vi "Tipo Señal.vi"(8 "error in (no error)":errorcluster, 10 "Tipo Señal":u16, 11 "F Generator in":refnum<class "F Generator.lvclass">) -> (0 "error out":errorcluster, 3 "F Generator out":refnum<class "F Generator.lvclass">)   [LabVIEW 2020, in "F Generator.lvlib" / "F Generator.lvclass"]
uses:
  F Generator.lvclass
  F Generator.lvclass/F Generator.ctl
  <vilib>/ActorFramework/Message Enqueuer/Message Enqueuer.lvclass/Message Enqueuer.ctl
  <vilib>/ActorFramework/Message Enqueuer/Enqueue.vi
  C:/Program Files/National Instruments/LabVIEW 2020/vi.lib/ActorFramework/Message/Message.lvclass
  <vilib>/ActorFramework/Message Priority Queue/Priority Enqueue.vi
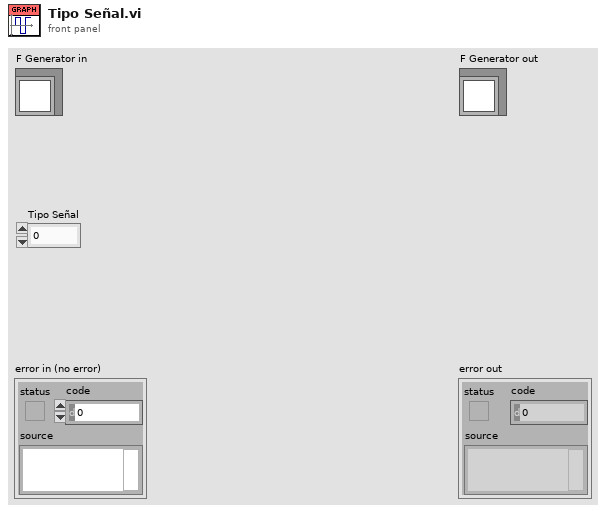
[diagram p1: front panel]
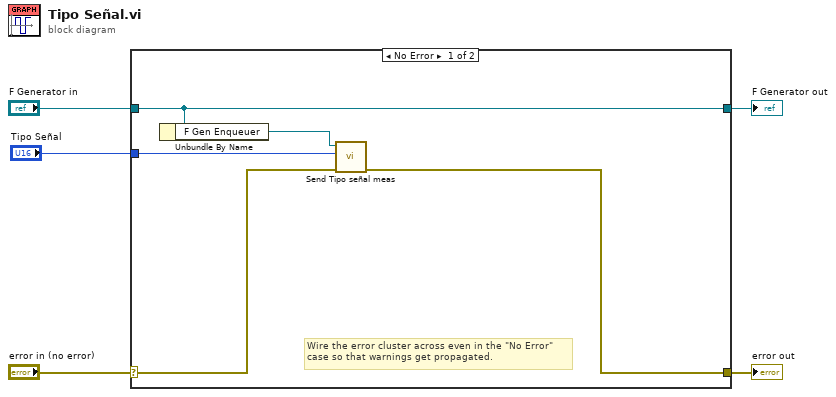
[diagram p0: block diagram]
diagram:
  n1 = case shown="No Error" "error in (no error)" {
    selector: "error in (no error)" -> [w7 w12]
    tunnel: [w6 w12] -> w4
    tunnel: [w10 w11] -> w2
    tunnel: "F Generator in" -> [w10 w11]
    tunnel: "Tipo Señal" -> [w8 _]
    frame No Error {
      # "Wire the error cluster across even in the \"No Error\"\ncase so that warnings get propagated."
      n2 = Unbundle By Name(w10) -> ("F Gen Enqueuer"=w9:refnum<class "Message Enqueuer.lvclass">)
      n3 = call "Send Tipo señal meas.vi"("error in (no error)"=w7, "Tipo Señal"=w8, "Message Enqueuer"=w9) -> ("error out"=w6:errorcluster)  [unwired: 7 in, 1 out]
    }
    frame Error {
    }
  }
  "error out" <- w4
  "F Generator out" <- w2
